vi "open another VI.vi"(11 "vi path":path) -> ()   [LabVIEW 2015]
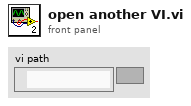
[diagram p1: front panel]
types:
  T1 = enum32{"Invalid", "Standard", "Closed", "Hidden", "Minimized", "Maximized"}
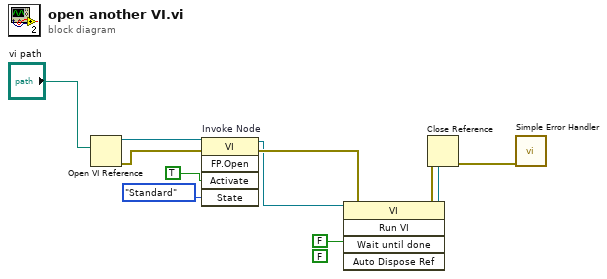
[diagram p0: block diagram]
diagram:
  (unwired) FALSE ("Auto Dispose Reference")
  n1 = Open VI Reference(vi path="vi path") -> (vi reference=w2:refnum<vi>, error out=w3:errorcluster)  [unwired: 1 in, 4 out]
  n2 = invoke on="Invoke Node" class="VI" method="FP.Open"(reference=w2, error in=w3, "Activate"=TRUE ("Activate?"), "State"=T1."Standard") -> (reference out=w7:refnum<vi>, error out=w8:errorcluster)  [unwired: 1 in, 3 out]
  n3 = invoke class="VI" method="Run VI"(reference=w7, error in=w8, "Wait until done"=FALSE ("Wait Until Done")) -> (reference out=w9:refnum<vi>, error out=w10:errorcluster)  [unwired: 2 in, 3 out]
  n4 = Close Reference(reference=w9, error in (no error)=w10) -> (error out=w4:errorcluster)
  n5 = call <vilib>:"Simple Error Handler.vi"("error in (no error)"=w4) -> ()  [unwired: 1 in, 8 out]
